vi "IntakeForTime.vi"() -> ()   [LabVIEW 2019]
uses:
  Framework/Robot Global Data.vi
panel:
  in  "NoWait":bool
  in  "Time":dbl
  in  "Speed":dbl
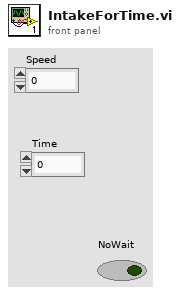
[diagram p1: front panel]
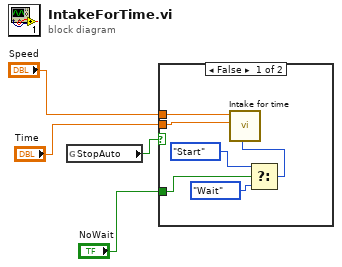
[diagram p0: block diagram]
diagram:
  n1 = global read "Robot Global Data.vi" "StopAuto"() -> (w4:bool)
  n2 = case shown="False" w4 {
    tunnel: "Speed" -> [w10 _]
    tunnel: "Time" -> [w9 _]
    tunnel: "NoWait" -> [w5 _]
    frame False {
      n3 = Select(t=enum16{"Start", "Wait"}."Start" ("Synchronization"), s=w5, f=enum16{"Start", "Wait"}."Wait" ("Synchronization")) -> (s? t:f=w6:enum16{"Start", "Wait"})
      n4 = call "Intake for time.vi"("Synchronization"=w6, "Duration (s)"=w9, "Setpoint"=w10) -> ()  [unwired: 8 in, 1 out]
    }
    frame True {
    }
  }
